vi "Write Item Name.vi"(8 "error in (no error)":errorcluster, 10 "Item Name":string, 11 "LabVIEWItem in":refnum<class "LabVIEWItem.lvclass">) -> (0 "error out":errorcluster, 3 "LabVIEWItem out":refnum<class "LabVIEWItem.lvclass">)   [LabVIEW 2019, in "Panther Dashboard.lvlib" / "LabVIEWItem.lvclass"]
uses:
  LabVIEWItem.lvclass
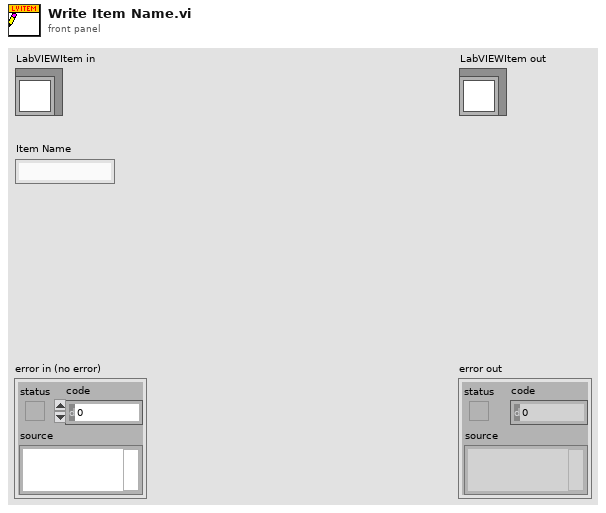
[diagram p1: front panel]
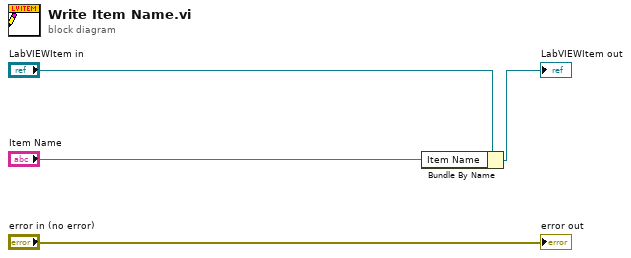
[diagram p0: block diagram]
diagram:
  n1 = Bundle By Name(cluster="LabVIEWItem in", "Item Name"="Item Name") -> (→"LabVIEWItem out":refnum<class "LabVIEWItem.lvclass">)
  "error out" <- "error in (no error)"
